vi "(21) part 2 que.vi"() -> ()   [LabVIEW 2025]
panel:
  in  "Y 2":dbl[](array[numeric])
  in  "waveform":waveform(dbl)
  in  "Y":dbl[](array[numeric])
  out "Waveform Graph 3":waveform(dbl)[](graph)
  out "Waveform Graph 2":dbl[][](graph)
  in  "Array 2":dbl[][](array[numeric])
  out "Waveform Graph":dbl[](graph)
  in  "Array":dbl[](array[numeric])
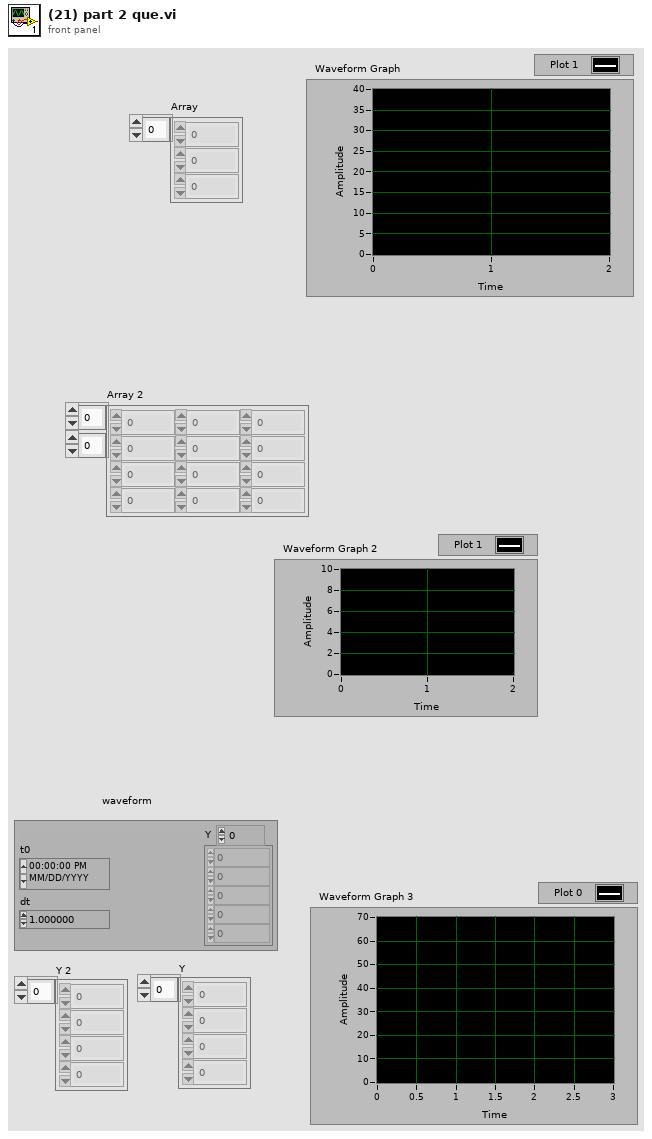
[diagram p1: front panel]
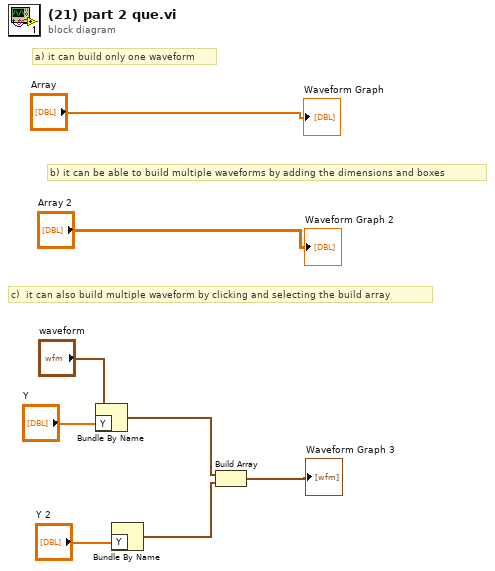
[diagram p0: block diagram]
diagram:
  # "c)  it can also build multiple waveform by clicking and selecting the build array"
  # "b) it can be able to build multiple waveforms by adding the dimensions and boxes"
  # "a) it can build only one waveform"
  n1 = Bundle By Name(cluster="waveform", "Y"="Y") -> (w3:waveform(dbl))
  n2 = Bundle By Name("Y"="Y 2") -> (w2:waveform(dbl))  [unwired: 1 in]
  n3 = Build Array(w3, w2) -> (→"Waveform Graph 3":waveform(dbl)[])
  "Waveform Graph" <- "Array"
  "Waveform Graph 2" <- "Array 2"
